vi "ExSimpleAsyncExampleGblQ.vi"() -> ()   [LabVIEW 2010]
uses:
  Open-Close/CamHandle.vi
panel:
  in  "Trigger Edge":u32(ring)=1 items=["N/A", "Positive (leading) edge", "Negative (falling) edge"]
  in  "Timing Mode":u32(ring)=1 items=["N/A", "Free Run/Timed", "Trigger First (PM only)", "Ext Sync/Strobed ", "Variable Exp (PM only)", "Flash Mode (PM only)"]
  in  "Temperature":dbl format="%.2f"
  in  "Exposure":dbl min=0.0 step=0.001 format="%.3f"
  in  "stop":bool
  in  "Store":bool
  out "error out":errorcluster
  in  "error in (no error)":errorcluster
  # "ExSimipleAsyncExample:\nThis is a Full Frame Async example. This should work with \nall camera systems. It requires a start for every frame \ncollected. Not all timing modes work for all cameras, also \nthe trigger edge only applies to Princeton Instrument \ncameras. Not all cameras have the ability to set the \ntemperature.\nPressing the stop button stops the example."
  # "NOTICE\n\nTHIS VI USES A GLOBAL CAMERA HANDLE\n\nTHE VI EXOPENGLOBALCAM.VI MUST BE\nRUN AT THE START OF THE WORK SESSION.\nTHE CAMERA WILL REMAIN OPENED.\n\nTHE VI EXCLOSEGLOBALCAM.VI MUST\nBE RUN BEFORE LEAVING LABVIEW."
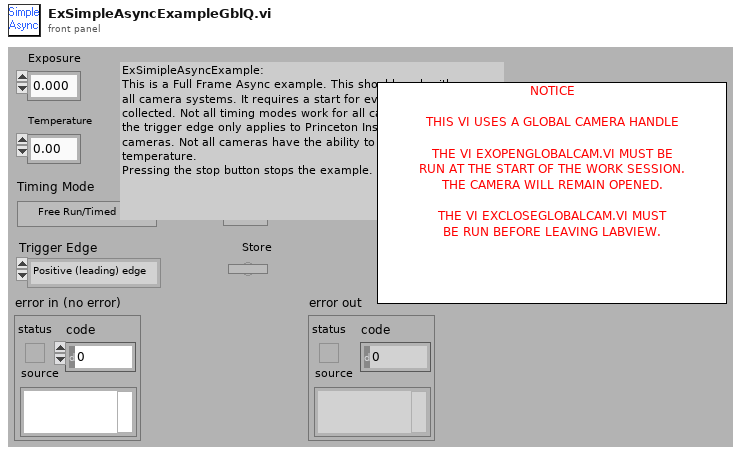
[diagram p1: front panel]
types:
  T1 = cluster{"Acquire mode \n3 is Async":i32, "Exposure":dbl, "Number of Images":i32, "Software Accums":i32}
  T2 = cluster{"Camera Handle":u32, "File Handle":u32, "Display Handle":u32, "Image Handle":u32}
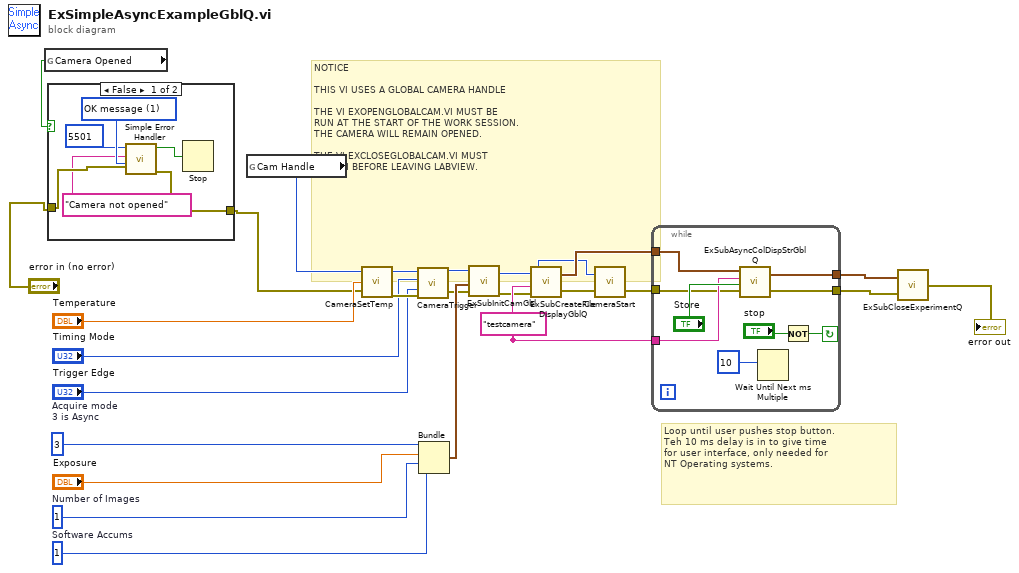
[diagram p0: block diagram]
diagram:
  w23 = 1  # Number of Images
  w24 = 3  # Acquire mode  3 is Async
  w22 = 1  # Software Accums
  w25 = "testcamera"
  # "NOTICE\n\nTHIS VI USES A GLOBAL CAMERA HANDLE\n\nTHE VI EXOPENGLOBALCAM.VI MUST BE\nRUN AT THE START OF THE WORK SESSION.\nTHE CAMERA WILL REMAIN OPENED.\n\nTHE VI EXCLOSEGLOBALCAM.VI MUST\nBE RUN BEFORE LEAVING LABVIEW."
  # "Loop until user pushes stop button.\nTeh 10 ms delay is in to give time \nfor user interface, only needed for \nNT Operating systems."
  n1 = global read "CamHandle.vi" "Camera Opened"() -> (w5:bool)
  n2 = case shown="False" w5 {
    tunnel: "error in (no error)" -> [w30 w32]
    tunnel: [w29 w32] -> w4
    frame False {
      w31 = u16 1 items=["no dialog", "OK message", "continue or stop message"] ("type of dialog (OK msg:1)")
      n3 = call <vilib>:"Simple Error Handler.vi"("error code (no error:0)"=5501, "error source (\" \")"="Camera not opened", "type of dialog (OK msg:1)"=w31, "error in (no error)"=w30) -> ("error?"=w27:bool, "error out"=w29:errorcluster)  [unwired: 1 in, 3 out]
      n4 = Stop(stop? (T)=w27) -> ()
    }
    frame True {
    }
  }
  n5 = global read "CamHandle.vi" "Cam Handle"() -> (w6:u32)
  n6 = call <userlib>:"CameraSetTemp.vi"("error in (no error)"=w4, "Temperature"="Temperature", "Camera Handle"=w6) -> ("error out"=w11:errorcluster, "Camera Handle"=w12:u32)
  n7 = call <userlib>:"CameraTrigger.vi"("error in"=w11, "Trigger Edge"="Trigger Edge", "Timing Mode"="Timing Mode", "Camera Handle"=w12) -> ("error out"=w8:errorcluster, "Camera Handle"=w7:u32)
  n8 = Bundle("Acquire mode \n3 is Async"=w24, "Exposure"="Exposure", "Number of Images"=w23, "Software Accums"=w22) -> (w20:T1)  [unwired: 1 in]
  n9 = call "ExSubInitCamGbl.vi"("error in (no error)"=w8, "Camera Information"=w20, "Camera Handle"=w7) -> ("error out"=w19:errorcluster, "Camera Handle"=w15:u32)
  n10 = call "ExSubCreateFileDisplayGblQ.vi"("error in (no error)"=w19, "File and Display Name"=w25, "Camera Handle"=w15) -> ("error out"=w18:errorcluster, "Handles Out"=w17:T2)  [unwired: 1 in]
  n11 = call <userlib>:"CameraStart.vi"("error in"=w18, "Camera Handle"=w15) -> ("error out"=w16:errorcluster)  [unwired: 1 out]
  n12 = while {
    tunnel: w17 -> [w33]
    tunnel: w16 -> [w38]
    tunnel: w25 -> [w39]
    tunnel: [w36] -> w2
    tunnel: [w37] -> w3
    stop <- w35 continue-if-true
    n13 = call "ExSubAsyncColDispStrGblQ.vi"("error in (no error)"=w38, "Store Data"="Store", "Display Title"=w39, "Handle Cluster"=w33) -> ("error out"=w36:errorcluster, "Handle Cluster Out"=w37:T2)
    n14 = Wait Until Next ms Multiple(millisecond multiple=10) -> ()  [unwired: 1 out]
    n15 = Not(x="stop") -> (.not. x?=w35:bool)
  }
  n16 = call "ExSubCloseExperimentQ.vi"("error in (no error)"=w2, "Handles In"=w3) -> ("error out"=→"error out":errorcluster)
